vi "Write Snake Status Remote.vi"(8 "error in (no error)":errorcluster, 11 "Snake in":refnum<class "Snake.lvclass">) -> (0 "error out":errorcluster, 3 "Snake out":refnum<class "Snake.lvclass">)   [LabVIEW 2021, in "Snake.lvclass"]
uses:
  Snake.lvclass
  Snake.lvclass/Snake.ctl
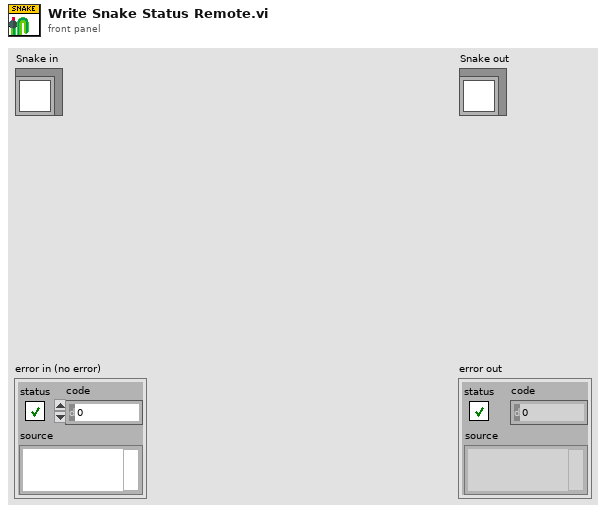
[diagram p1: front panel]
types:
  T1 = typedef "Snake.lvclass/Snake Status.ctl" = cluster{"Boosters":cluster{"Shield":bool, "Star":bool}, "Weakeners":cluster{"Grapes":bool, "Bomb Crash":bool, "Death":bool}}
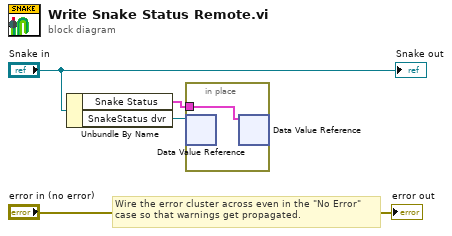
[diagram p0: block diagram]
diagram:
  # "Wire the error cluster across even in the \"No Error\"\ncase so that warnings get propagated."
  n1 = Unbundle By Name("Snake in") -> ("Snake Status"=w1:T1, "SnakeStatus dvr"=w2:refnum<data-value>)
  n2 = in-place {
    in-place-border: w1 -> [w5]
    n3 = in-place-dvr #1(w2) -> ()  [unwired: 2 out]
    n4 = in-place-dvr #1(w5) -> ()  [unwired: 2 out]
  }
  "error out" <- "error in (no error)"
  "Snake out" <- "Snake in"
